vi "Read Replace Default SPI Engine_.vi"(8 "error in (no error)":errorcluster, 11 "Bus Configuration in":refnum<class "Bus Configuration.lvclass">) -> (0 "error out":errorcluster, 2 "Replace Default SPI Engine?":bool, 3 "Bus Configuration out":refnum<class "Bus Configuration.lvclass">)   [LabVIEW 2014, in "Bus Configuration.lvclass"]
uses:
  Bus Configuration.lvclass
  Bus Configuration.lvclass/Bus Configuration.ctl
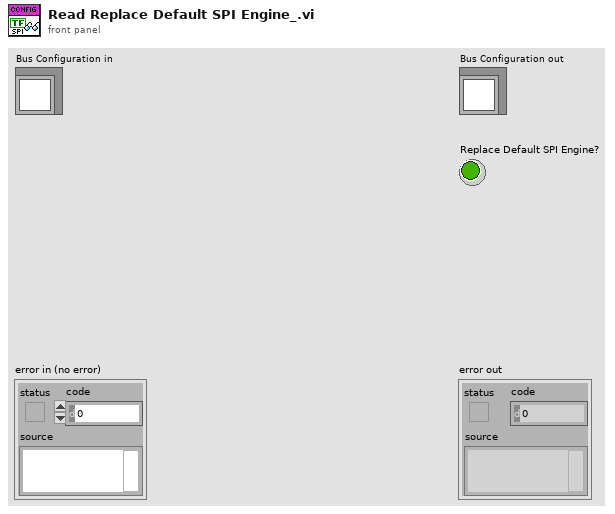
[diagram p1: front panel]
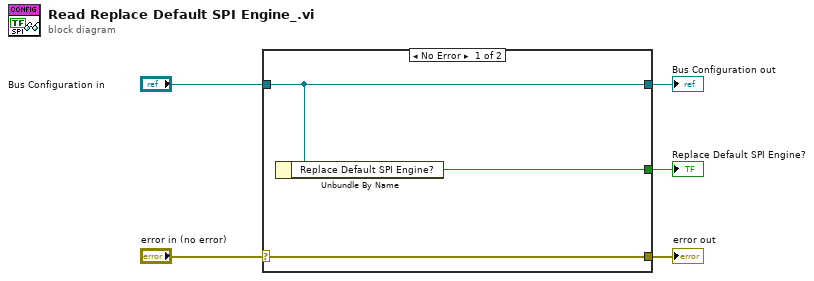
[diagram p0: block diagram]
diagram:
  n1 = case shown="No Error" "error in (no error)" {
    selector: "error in (no error)" -> [w8 w9]
    tunnel: [w8 w9] -> w4
    tunnel: [w7 w10] -> w2
    tunnel: "Bus Configuration in" -> [w7 w10]
    tunnel: [w6 _] -> w1
    frame No Error {
      n2 = Unbundle By Name(w7) -> ("Replace Default SPI Engine?"=w6:bool)
    }
    frame Error {
    }
  }
  "error out" <- w4
  "Bus Configuration out" <- w2
  "Replace Default SPI Engine?" <- w1
